vi "PCA9525 - Write.vi"(8 "error in (no error)":errorcluster, 9 "buffer":u8[](array[numeric])=[6, 0, 0], 10 "deviceAddress":u8=32 format="%x", 11 "handle":u64 format="%x") -> (0 "error out":errorcluster, 1 "sizeTransferred (Output)":u32, 2 "return (Output)":u64, 3 "handle 2":u64)   [LabVIEW 2024]
doc: "C command for writing to the PCA9535 using I2C."
uses:
  Users/Test Eng/Desktop/RIB Box - I2C - LabVIEW - Estops/RIB_Box_I2C_Estops/libmpsse.dll
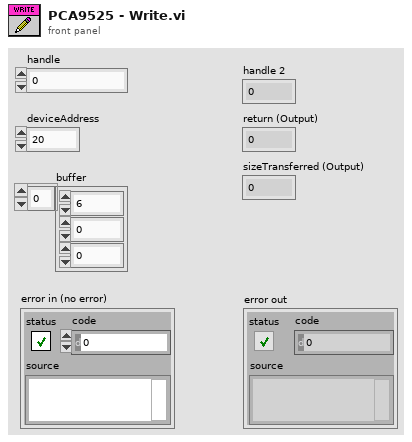
[diagram p1: front panel]
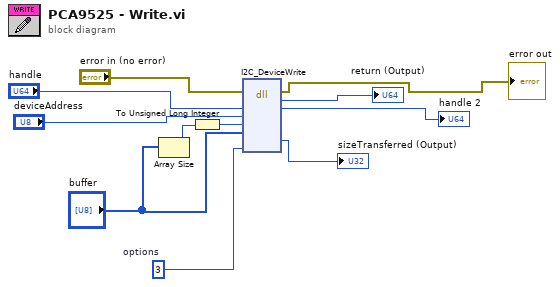
[diagram p0: block diagram]
diagram:
  w9 = u32 3  # options
  n1 = Array Size(array="buffer") -> (size(s)=w1:i32)
  n2 = To Unsigned Long Integer(number=w1) -> (unsigned 32bit integer=w2:u32)
  n3 = dll-call lib="C:/Users/Test Eng/Desktop/RIB Box - I2C - LabVIEW - Estops/RIB_Box_I2C_Estops/libmpsse.dll" fn="I2C_DeviceWrite"(error in="error in (no error)", "handle"="handle", "deviceAddress"="deviceAddress", "sizeToTransfer"=w2, "buffer"="buffer", "options"=w9) -> (error out=→"error out":errorcluster, "return type"=→"return (Output)":u64, "handle"=→"handle 2":u64, "sizeTransferred"=→"sizeTransferred (Output)":u32)  [unwired: 7 in, 1 out]
